vi "CLI Pre-Build Action.vi"(6 "Top Level/Always Included VIs":path[](array[path]), 7 "Main Destination Path":path, 9 "Target Name":string, 10 "Build Specification Name":string, 11 "Project Path":path) -> (0 "error out":errorcluster)   [LabVIEW 2020, in "GPackBuildSupport.lvlib"]
uses:
  GPackBuildSupport.lvlib
  <vilib>/Utility/traverseref.llb/TRef TravTarget.ctl
  GPack/Package/Package.lvclass
  GPackTools/CLIAction/CLIAction.lvclass
  <vilib>/Utility/miscctls.llb/LVPointTypeDef.ctl
  GPack/Build Cubedrop.vi
  GPack/GPack.lvlib
  <vilib>/Utility/traverseref.llb/VI Scripting - Traverse.lvlib
  <vilib>/Utility/EditLVProj/Edit LVProj.lvlib
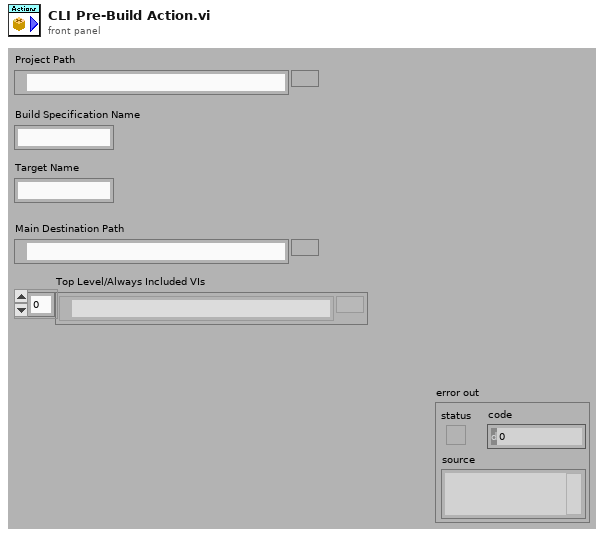
[diagram p1: front panel]
types:
  T1 = typedef "TRef TravTarget.ctl" = enum16{"FP", "BD", "Other"}
  T2 = typedef "Edit LVProj.lvlib/Library And VI References.ctl" = cluster{"Target Reference":refnum<vi>, "VI References":refnum<vi>[], "Library References":refnum<vi>[]}
  T3 = typedef "LVPointTypeDef.ctl" = cluster{"Horizontal":i16, "Vertical":i16}
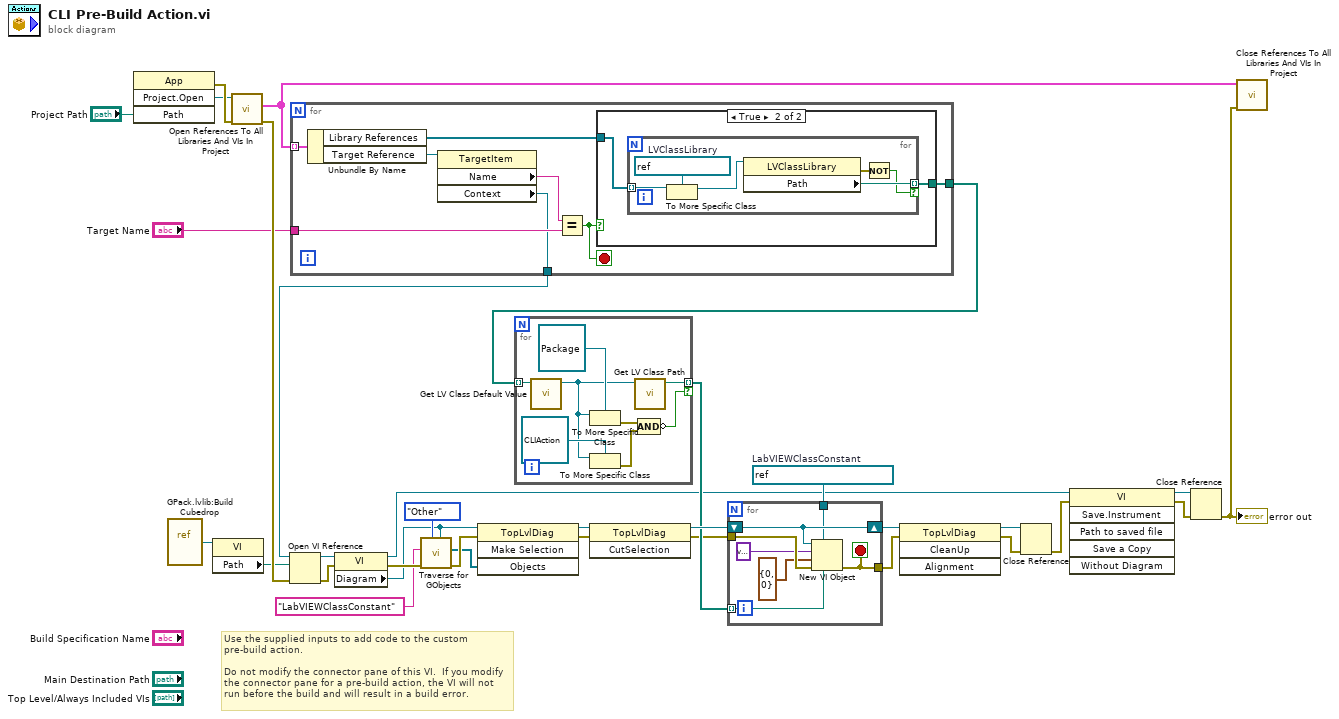
[diagram p0: block diagram]
diagram:
  w16 = refnum<vi> refnum  # LabVIEWClassConstant
  # "Use the supplied inputs to add code to the custom pre-build action.\n\nDo not modify the connector pane of this VI.  If you modify the connector pane for a pre-build action, the VI will not run before the build and will result in a build error."
  n1 = invoke class="App" method="Project.Open"("Path"="Project Path") -> (error out=w32:errorcluster, "Project:Open"=w6:refnum<vi>)  [unwired: 3 in, 2 out]
  n2 = vi-ref "GPack.lvlib:Build Cubedrop.vi"() -> (w28:refnum<vi>)
  n3 = property class="VI"(reference=w28) -> ("Path"=w27:path)  [unwired: 1 in, 2 out]
  n4 = call <vilib>:"Open References To All Libraries And VIs In Project.vi"("error in (no error)"=w32, "Project in"=w6) -> ("error out"=w33:errorcluster, "VI and Library References"=w1:T2[])  [unwired: 7 in, 1 out]
  n5 = for {
    tunnel: w1 -> [w41] mode=indexing
    tunnel: "Target Name" -> [w38]
    tunnel: [w36] -> w4
    tunnel: [w34] -> w3
    stop <- w35 stop-if-true
    n6 = Unbundle By Name(w41) -> ("Library References"=w37:refnum<vi>[], "Target Reference"=w40:refnum<vi>)
    n7 = property class="TargetItem"(reference=w40) -> ("Name"=w39:string, "Context"=w34:refnum<vi>)  [unwired: 1 in, 2 out]
    n8 = Equal?(x=w39, y=w38) -> (x = y?=w35:bool)
    n9 = case shown="True" w35 {
      tunnel: w37 -> [_ w43]
      tunnel: [_ w42] -> w36
      frame False {
      }
      frame True {
        n10 = for {
          tunnel: w43 -> [w49] mode=indexing
          tunnel: [w46] -> w42 mode=indexing if=w44
          w48 = refnum<vi> refnum  # LVClassLibrary
          n11 = To More Specific Class(target class=w48, reference=w49) -> (specific class reference=w47:refnum<vi>)  [unwired: 1 in, 1 out]
          n12 = property class="LVClassLibrary"(reference=w47) -> (error out=w45:errorcluster, "Path"=w46:path)  [unwired: 1 in, 1 out]
          n13 = Not(x=w45) -> (.not. x?=w44:bool)
        }
      }
    }
  }
  n14 = Open VI Reference(application reference (local)=w3, vi path=w27, error in (no error)=w33) -> (vi reference=w23:refnum<vi>, error out=w22:errorcluster)  [unwired: 3 in]
  n15 = property class="VI"(reference=w23, error in=w22) -> (reference out=w10:refnum<vi>, error out=w31:errorcluster, "Diagram"=w21:refnum<vi>)
  n16 = call <vilib>:"Traverse for GObjects.vi"("Other Refnum"=w21, "Traverse Target"=TRef_TravTarget."Other", "error in (no error)"=w31, "Class Name"="LabVIEWClassConstant") -> ("error out"=w30:errorcluster, "References"=w24:refnum<vi>[])  [unwired: 4 in, 2 out]
  n17 = invoke class="TopLvlDiag" method="Make Selection"(reference=w21, error in=w30, "Objects"=w24) -> (reference out=w20:refnum<vi>, error out=w19:errorcluster)  [unwired: 1 in, 2 out]
  n18 = for {
    tunnel: [w51] -> w17 mode=indexing if=w53
    tunnel: w4 -> [w50] mode=indexing
    n19 = call <vilib>:"Get LV Class Default Value.vi"("class path"=w50) -> ("object"=w52:refnum<class>)  [unwired: 9 in, 1 out]
    n20 = To More Specific Class(target class=refnum<class "Package.lvclass"> refnum ("GPack.lvlib:Package.lvclass"), reference=w52) -> (error out=w55:errorcluster)  [unwired: 1 in, 1 out]
    n21 = To More Specific Class(target class=refnum<class "CLIAction.lvclass"> refnum ("GPackTools.lvlib:CLIAction.lvclass"), reference=w52) -> (error out=w54:errorcluster)  [unwired: 1 in, 1 out]
    n22 = call <vilib>:"Get LV Class Path.vi"("object"=w52) -> ("class path"=w51:path)  [unwired: 9 in, 1 out]
    n23 = Compound Arithmetic op=AND(w55, w54) -> (invert w53:bool)
  }
  n24 = invoke class="TopLvlDiag" method="CutSelection"(reference=w20, error in=w19) -> (reference out=w18:refnum<vi>, error out=w15:errorcluster)  [unwired: 1 in, 1 out]
  n25 = for {
    shift-right: [w62] -> w14
    shift-left: w18 -> [w62]
    tunnel: w17 -> [w63] mode=indexing
    tunnel: w16 -> [w59]
    tunnel: w15 -> [w64]
    tunnel: [w58] -> w13
    stop <- w58 stop-if-true
    n26 = New VI Object(vi object class=w59, owner refnum=w62, style=variant, position/next to=T3 {"Horizontal"=0, "Vertical"=0} ("location"), 6:w63, 8:w64) -> (0:w58:errorcluster)  [unwired: 2 in, 1 out]
  }
  n27 = invoke class="TopLvlDiag" method="CleanUp"(reference=w14, error in=w13) -> (reference out=w12:refnum<vi>, error out=w11:errorcluster)  [unwired: 2 in, 2 out]
  n28 = Close Reference(reference=w12, error in (no error)=w11) -> (error out=w9:errorcluster)
  n29 = invoke class="VI" method="Save.Instrument"(reference=w10, error in=w9) -> (reference out=w7:refnum<vi>, error out=w8:errorcluster)  [unwired: 4 in, 4 out]
  n30 = Close Reference(reference=w7, error in (no error)=w8) -> (error out=w2:errorcluster)
  "error out" <- w2
  n31 = call <vilib>:"Close References To All Libraries And VIs In Project.vi"("error in (no error)"=w2, "VI and Library References"=w1) -> ()  [unwired: 9 in, 1 out]
